vi "ABB Select configure 2.vi"() -> ()   [LabVIEW 2017]
panel:
  in  "Efficiencies":bool
  in  "Bearing run":bool
  in  "Locked rotor":bool
  in  "No Load":bool
  in  "Temperatures":bool
  in  "Heat Run":bool
  in  "Exit":bool
  # "Configure"
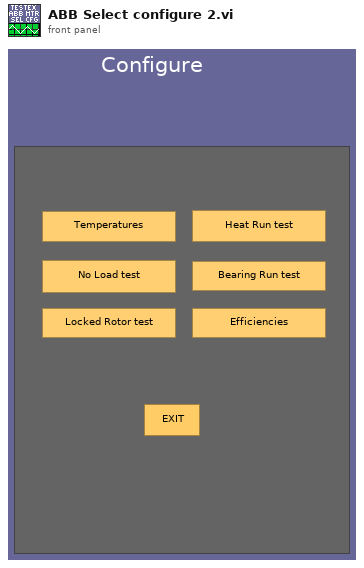
[diagram p1: front panel]
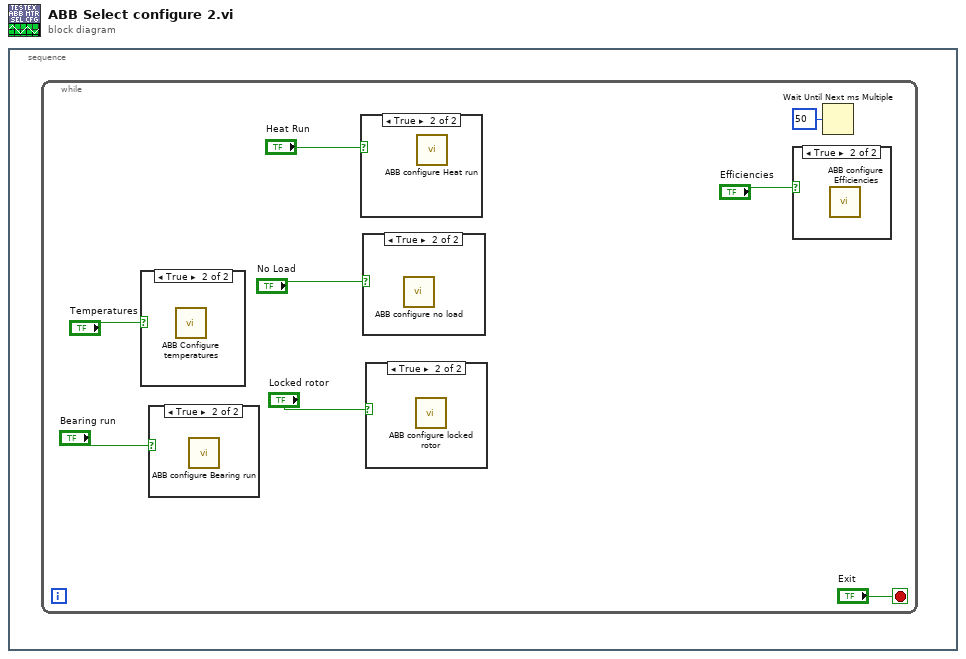
[diagram p0: block diagram]
diagram:
  n1 = stacked-sequence {
    frame #0 {
      n2 = while {
        stop <- "Exit" stop-if-true
        n3 = case shown="True" "Temperatures" {
          frame False {
          }
          frame True {
            n4 = call "ABB Configure temperatures.vi"() -> ()  [unwired: 1 in]
          }
        }
        n5 = case shown="True" "Bearing run" {
          frame False {
          }
          frame True {
            n6 = call "ABB configure Bearing run.vi"() -> ()  [unwired: 1 in]
          }
        }
        n7 = case shown="True" "Heat Run" {
          frame False {
          }
          frame True {
            n8 = call "ABB configure Heat run.vi"() -> ()  [unwired: 1 in]
          }
        }
        n9 = case shown="True" "No Load" {
          frame False {
          }
          frame True {
            n10 = call "ABB configure no load.vi"() -> ()  [unwired: 1 in]
          }
        }
        n11 = case shown="True" "Locked rotor" {
          frame False {
          }
          frame True {
            n12 = call "ABB configure locked rotor.vi"() -> ()  [unwired: 1 in]
          }
        }
        n13 = case shown="True" "Efficiencies" {
          frame False {
          }
          frame True {
            n14 = call "ABB configure Efficiencies.vi"() -> ()  [unwired: 1 in]
          }
        }
        n15 = Wait Until Next ms Multiple(millisecond multiple=u32 50) -> ()  [unwired: 1 out]
      }
    }
  }
